vi "SecondFunPj.vi"() -> ()   [LabVIEW 2012]
panel:
  in  "stop":bool
  out "Numeric 3":dbl
  in  "Numeric 2":dbl
  in  "Numeric":dbl
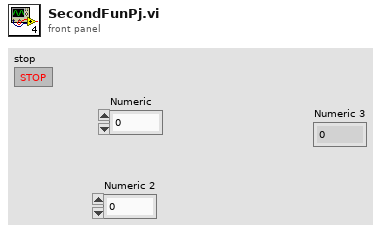
[diagram p1: front panel]
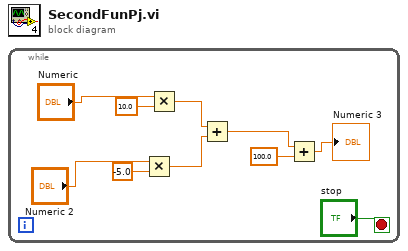
[diagram p0: block diagram]
diagram:
  n1 = while {
    stop <- "stop" stop-if-true
    n2 = Multiply(x="Numeric 2", y=-5.0) -> (x*y=w4:dbl)
    n3 = Multiply(x="Numeric", y=10.0) -> (x*y=w5:dbl)
    n4 = Add(x=w5, y=w4) -> (x+y=w3:dbl)
    n5 = Add(x=w3, y=100.0) -> (x+y=→"Numeric 3":dbl)
  }
